vi "Global Control Outputs.vi"() -> ()   [LabVIEW 2017, in "Controller.lvlib"]
uses:
  Controller.lvlib
panel:
  out "Strafe Right":bool
  out "Strafe Left":bool
  out "Override":bool
  out "Enable Shooter Overlord":bool
  out "Rotate Right":bool
  out "Rotate  Left":bool
  out "Decrease Shooter RPM":bool
  out "Increase Shooter RPM":bool
  out "Decrement Hood":bool
  out "Increment Hood":bool
  out "Jam Release":bool
  out "Switch View":bool
  in  "Motion Buttons Output":u16 format="%04x"
  out "Intake On":bool
  out "Reset Gyro":bool
  out "Snap To Blue Retrieval Station":bool
  out "Snap To Red Retrieval Station":bool
  out "Snap To Blue Boiler":bool
  out "Snap To Red Boiler":bool
  out "Turn Left 90":bool
  out "Turn Right 90":bool
  out "Snap To Right Rope":bool
  out "Snap To Left Rope":bool
  out "Snap To Right Peg":bool
  out "Snap To Left Peg":bool
  out "Snap To 180":bool
  out "Snap To 0":bool
  out "Climb":bool
  out "Abort":bool
  out "Place Gear":bool
  out "Fire!":bool
  out "Prepare to Shoot":bool
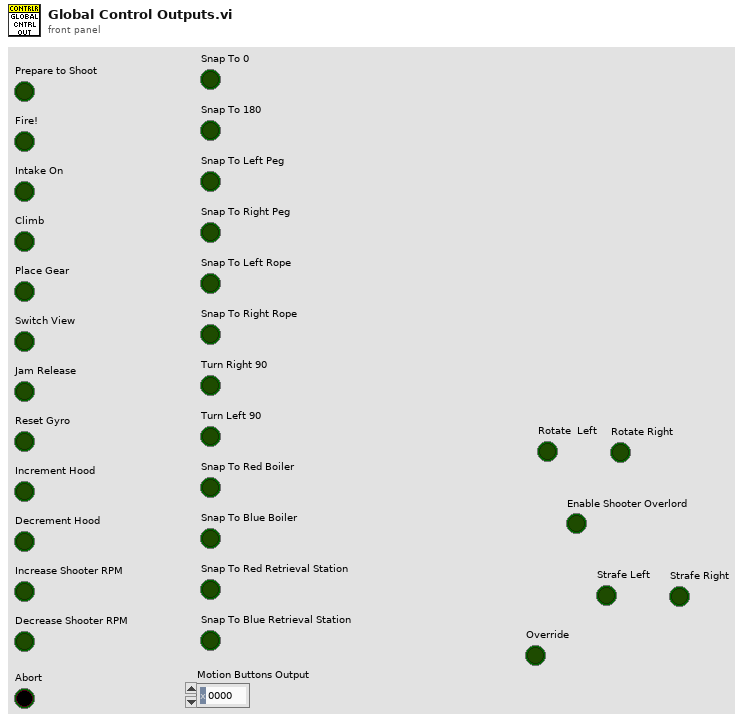
[diagram p1: front panel]
diagram:
